vi "Assemble Process Builder ViewManager.vi"(9 "Main ViewManager":refnum<class "Main ViewManager.lvclass">, 10 "Process Builder ViewManager":refnum<class "Test Executive Builder ViewManager.lvclass">, 11 "Navigation View.lvclass":refnum<class "Navigation View.lvclass">) -> (3 "Main ViewManager out":refnum<class "Navigation ViewManager.lvclass">)   [LabVIEW 2020, in "Navigation ViewManager.lvclass"]
uses:
  <vilib>/gpm_packages/@cs/Car-wash/Source/Process Builder ViewManager/Navigation ViewManager.lvclass
  C:/Program Files/National Instruments/LabVIEW 2020/vi.lib/gpm_packages/@cs/mva-viewable/Source/IViewManager/IViewManager/IViewManager.lvclass
  <vilib>/gpm_packages/@cs/Test-executive-builder/Source/Test Executive Builder ViewManager/Test Executive Builder ViewManager/Test Executive Builder ViewManager.lvclass
  C:/Program Files/National Instruments/LabVIEW 2020/vi.lib/gpm_packages/@cs/mva-viewable/Source/IViewable/IViewable/IViewable.lvclass
  <vilib>/gpm_packages/@cs/Car-wash/Source/Main ViewManager/Main ViewManager/Main ViewManager.lvclass
  <vilib>/gpm_packages/@cs/Car-wash/Source/Navigation View/Navigation View.lvclass
  <vilib>/gpm_packages/@cs/mva-viewable/Source/IViewManager/IViewManager Messages/Launch Nested Views Msg/Launch Nested Views Msg.lvclass/Launch Nested Views Msg.ctl
  <vilib>/gpm_packages/@cs/mva-viewable/Source/IViewManager/IViewManager/IViewManager.lvclass/IViewManager.ctl
  <vilib>/gpm_packages/@cs/mva-viewable/Source/IViewManager/IViewManager Messages/Launch Nested Views Msg/Pack Launch Nested Views Msg.vi
  <vilib>/gpm_packages/@cs/mva-viewable/Source/IViewManager/IViewManager Messages/Launch Nested Views Msg/Launch Nested Views Msg.lvclass
  <vilib>/gpm_packages/@cs/mva-viewable/Source/IViewManager/IViewManager/IViewManager.lvclass
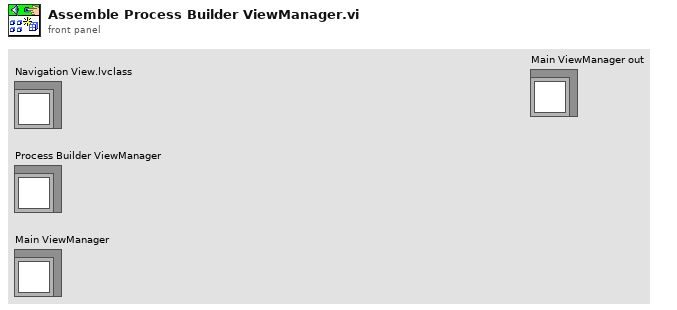
[diagram p1: front panel]
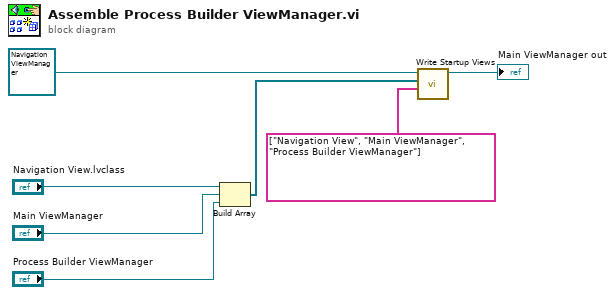
[diagram p0: block diagram]
diagram:
  n1 = Build Array("Navigation View.lvclass", "Main ViewManager", "Process Builder ViewManager") -> (w1:refnum<class "IViewable.lvclass">[])
  n2 = call <vilib>:"Write Startup Views.vi"("View Labels"=string[] ["Navigation View", "Main ViewManager", "Process Builder ViewManager"], "Startup Views"=w1, "IViewManager in"=refnum<class "Navigation ViewManager.lvclass"> refnum ("Main ViewManager.lvlib:Main ViewManager.lvclass")) -> ("IViewManager out"=→"Main ViewManager out":refnum<class "Navigation ViewManager.lvclass">)  [unwired: 8 in]
